vi "Switch Configuration - Filter Mux Models.vi"(8 "error in (no error)":errorcluster, 11 "Switch Config UI Data In":T1 {"Switch Config Page Item Ref" format="%.0x"}) -> (0 "error out":errorcluster, 2 "First Mux Model":string, 3 "Switch Config UI Data Out":T1 {"Switch Config Page Item Ref" format="%.0x"})   [LabVIEW 2015, in "DMM-SWITCH-ScanList System Explorer.lvlib"]
doc: "Get supported Mux Models from supported Mux Topologies Array. Update the Switch Model ComboBox with the generated array."
uses:
  DMM-SWITCH-ScanList System Explorer.lvlib
  Configuration Controls/Switch Config VI UI Data.ctl
  Configuration Controls/Switch Config VI UI Ctrl Values.ctl
  Configuration Controls/Switch Config VI UI Ctrl References.ctl
  <instrlib>/niSwitch/niSwitch.LLB/niSwitch Topologies.ctl
  <vilib>/NI Veristand/Custom Device API/Custom Device Item Ref.ctl
  <vilib>/NI Veristand/Custom Device API/Custom Device API.lvlib
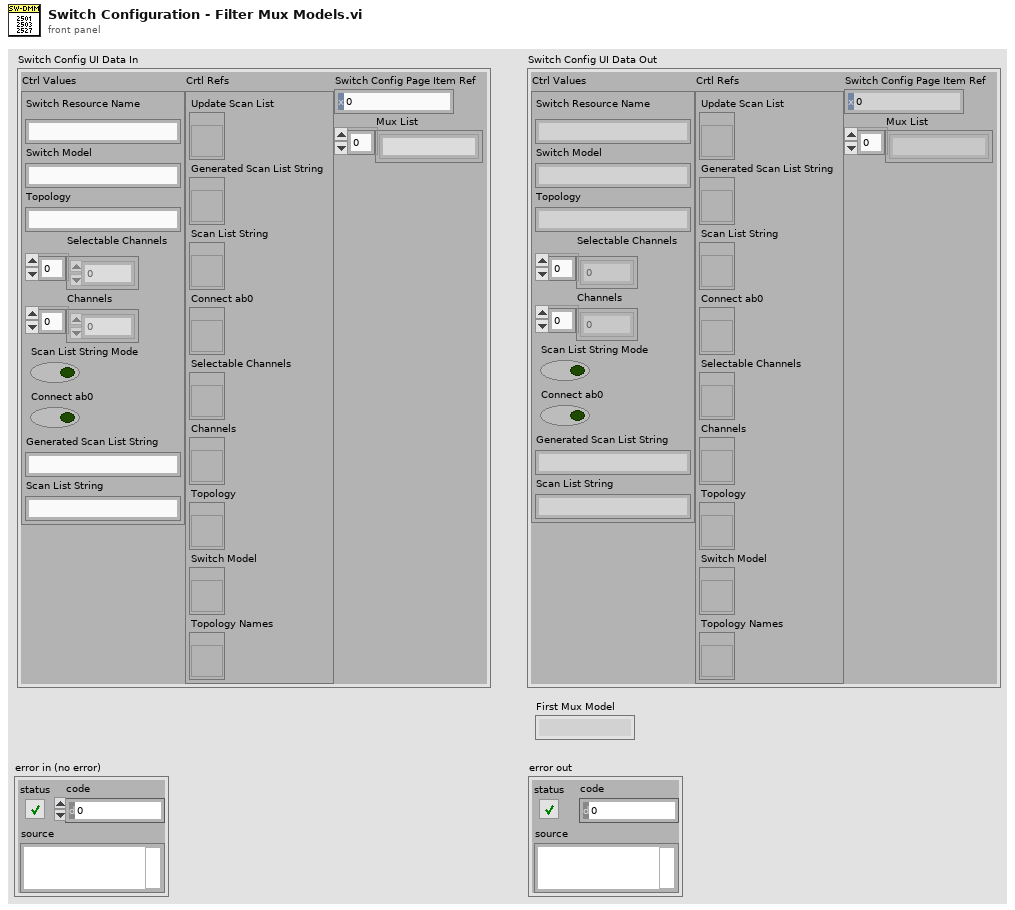
[diagram p1: front panel]
types:
  T1 = typedef "DMM-SWITCH-ScanList System Explorer.lvlib/Switch Config VI UI Data.ctl" = cluster{"Ctrl Values":T2, "Crtl Refs":T3, "Switch Config Page Item Ref":T4, "Mux List":string[]}
  T2 = typedef "DMM-SWITCH-ScanList System Explorer.lvlib/Switch Config VI UI Ctrl Values.ctl" = cluster{"Switch Resource Name":string, "Switch Model":string, "Topology":string, "Selectable Channels":i32[], "Channels":i32[], "Scan List String Mode":bool, "Connect ab0":bool, "Generated Scan List String":string, "Scan List String":string}
  T3 = typedef "DMM-SWITCH-ScanList System Explorer.lvlib/Switch Config VI UI Ctrl References.ctl" = cluster{"Update Scan List":refnum<vi>, "Generated Scan List String":refnum<vi>, "Scan List String":refnum<vi>, "Connect ab0":refnum<vi>, "Selectable Channels":refnum<vi>, "Channels":refnum<vi>, "Topology":refnum<vi>, "Switch Model":refnum<vi>, "Topology Names":refnum<vi>}
  T4 = typedef "Custom Device API.lvlib/Custom Device Item Ref.ctl" = u64
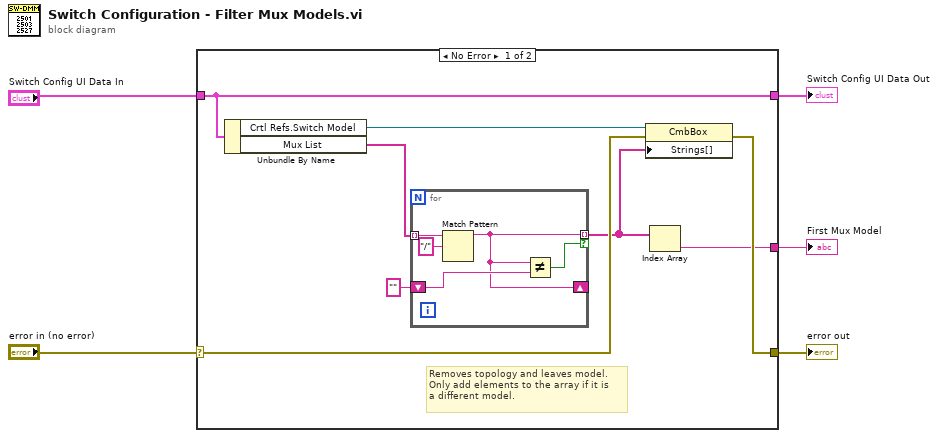
[diagram p0: block diagram]
diagram:
  n1 = case shown="No Error" "error in (no error)" {
    selector: "error in (no error)" -> [w11 w20]
    tunnel: [w13 w20] -> w5
    tunnel: "Switch Config UI Data In" -> [w6 w19]
    tunnel: [w12 _] -> w4
    tunnel: [w6 w19] -> w1
    frame No Error {
      # "Removes topology and leaves model.\nOnly add elements to the array if it is\na different model."
      n2 = Unbundle By Name(w6) -> ("Crtl Refs.Switch Model"=w8:refnum<vi>, "Mux List"=w7:string[])
      n3 = for {
        tunnel: w7 -> [w18] mode=indexing
        tunnel: [w15] -> w10 mode=indexing if=w14
        shift-right: [w15] -> _
        shift-left: "" -> [w16]
        n4 = Match Pattern(string=w18, regular expression="/") -> (before substring=w15:string)  [unwired: 1 in, 3 out]
        n5 = Not Equal?(x=w15, y=w16) -> (x != y?=w14:bool)
      }
      n6 = property class="CmbBox"(reference=w8, error in=w11, "Strings[]"=w10) -> (error out=w13:errorcluster)  [unwired: 1 out]
      n7 = Index Array(array=w10) -> (element=w12:string)  [unwired: 1 in]
    }
    frame Error {
    }
  }
  "error out" <- w5
  "First Mux Model" <- w4
  "Switch Config UI Data Out" <- w1
